vi "Break In 16x32 Bit Chunks.vi"(11 "2D Nx512 Array":bool[](array[boolean])) -> (3 "Array":bool[][](array[boolean]))   [LabVIEW 2014]
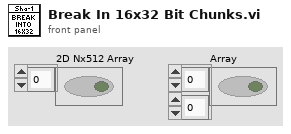
[diagram p1: front panel]
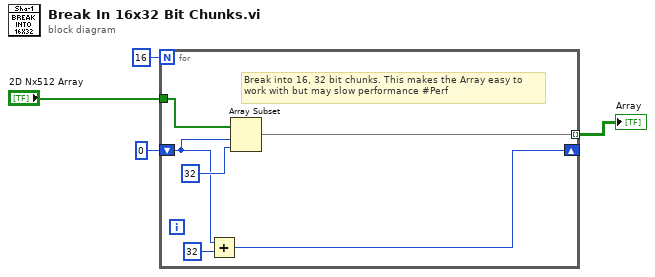
[diagram p0: block diagram]
diagram:
  n1 = for {
    N: 16 -> [_]
    tunnel: "2D Nx512 Array" -> [w10]
    shift-right: [w6] -> _
    shift-left: 0 -> [w7]
    tunnel: [w5] -> w3 mode=indexing
    # "Break into 16, 32 bit chunks. This makes the Array easy to\nwork with but may slow performance #Perf"
    n2 = Add(x=w7, y=32) -> (x+y=w6:i32)
    n3 = Array Subset(array=w10, index=w7, length=32) -> (w5:bool[])
  }
  "Array" <- w3
